vi "Sudo Wrapper.vi"(7 "Install LV Data":T1={"SSH Session"=refnum, "Status Log"="", "Detailed Log"="", "Credentials"={"Hostname or IP"="192.168.7.2", "Username"="root", "Password"=""}, "Target Info"={"OS Version"="", "CPU"="", "Systemd Version"="", "Internet Access"=FALSE, "Device Type"="", "LV Installed Ver"="", "LV Available Ver"="", "LV Upgrade Available"=FALSE, "Hostname"="", "NIC Info"=[]}, "Reboot Required?"=FALSE}, 9 "comand string":string, 11 "echo string":string) -> (3 "combined command string":string)   [LabVIEW 2020, in "LMH-LINX.lvlib"]
uses:
  LMH-LINX.lvlib
  Target Management/Install LV Data.ctl
  Target Management/Target Info.ctl
  Target Management/NIC Info.ctl
  Target Management/NIC Mode.ctl
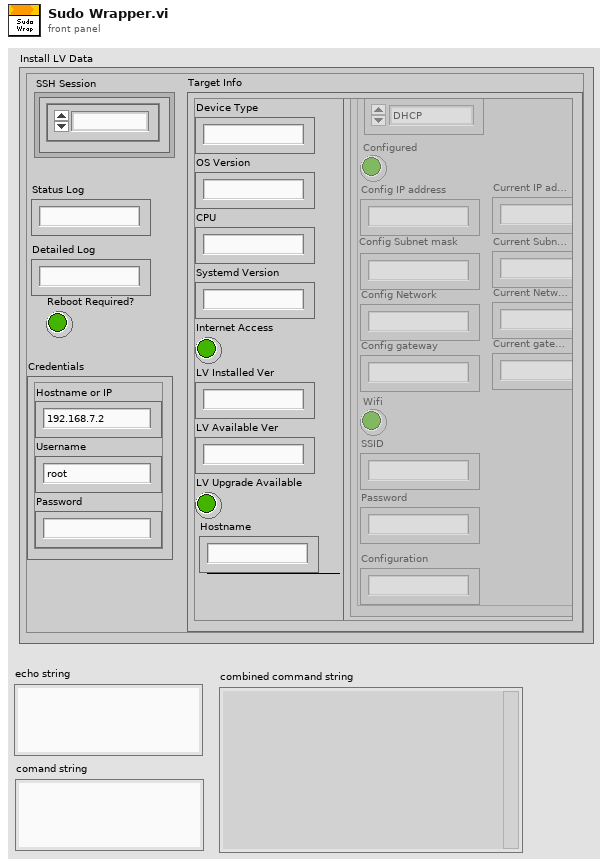
[diagram p1: front panel]
types:
  T1 = typedef "LMH-LINX.lvlib/Install LV Data.ctl" = cluster{"SSH Session":refnum<k1>, "Status Log":string, "Detailed Log":string, "Credentials":cluster{"Hostname or IP":string, "Username":string, "Password":string}, "Target Info":T2, "Reboot Required?":bool}
  T2 = typedef "LMH-LINX.lvlib/Target Info.ctl" = cluster{"OS Version":string, "CPU":string, "Systemd Version":string, "Internet Access":bool, "Device Type":string, "LV Installed Ver":string, "LV Available Ver":string, "LV Upgrade Available":bool, "Hostname":string, "NIC Info":T3[]}
  T3 = typedef "LMH-LINX.lvlib/NIC Info.ctl" = cluster{"Name":string, "NIC Mode":T4, "Configured":bool, "Config IP address":string, "Config Subnet mask":string, "Config Network":string, "Config gateway":string, "Wifi":bool, "SSID":string, "Password":string, "Configuration":string, "Current IP address":string, "Current Subnet mask":string, "Current gateway":string, "Current Network":string}
  T4 = typedef "LMH-LINX.lvlib/NIC Mode.ctl" = enum16{"DHCP", "Static", "Loopback"}
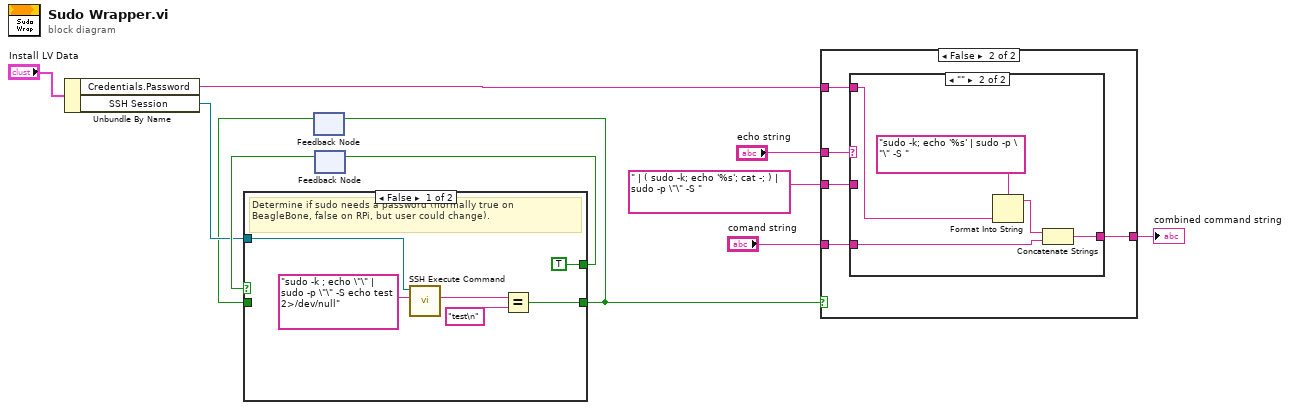
[diagram p0: block diagram]
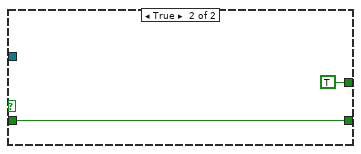
[diagram p2: hidden frame]
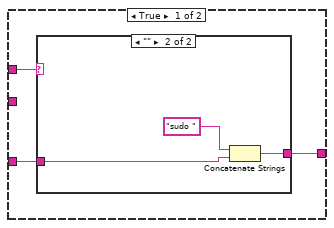
[diagram p3: hidden frame]
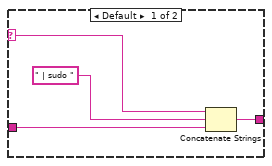
[diagram p4: hidden frame]
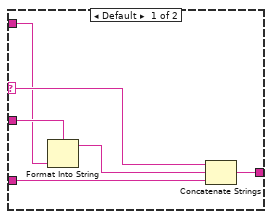
[diagram p5: hidden frame]
diagram:
  n1 = Unbundle By Name("Install LV Data") -> ("Credentials.Password"=w6:string, "SSH Session"=w3:refnum<k1>)
  n2 = feedback #1() -> (w2:bool)  [unwired: 1 in]
  n3 = feedback #2() -> (w5:bool)  [unwired: 1 in]
  n4 = case shown="False" w5 {
    tunnel: [TRUE TRUE] -> w4
    tunnel: w3 -> [w15 _]
    tunnel: [w12 w19] -> w1
    tunnel: w2 -> [_ w19]
    frame False {
      # "Determine if sudo needs a password (normally true on\nBeagleBone, false on RPi, but user could change)."
      n5 = call "SSH Execute Command.vi"("Command"="sudo -k ; echo \"\" | sudo -p \"\" -S echo test  2>/dev/null", "SSH Session"=w15) -> ("Std Out"=w14:string)  [unwired: 7 in, 2 out]
      n6 = Equal?(x=w14, y="test\n") -> (x = y?=w12:bool)
    }
    frame True {
    }
  }
  n7 = feedback-in #1(w1) -> ()
  n8 = feedback-in #2(w4) -> ()
  n9 = case shown="False" w1 {
    tunnel: "echo string" -> [w21 w34]
    tunnel: "comand string" -> [w20 w33]
    tunnel: [w22 w32] -> w9
    tunnel: " | ( sudo -k; echo '%s'; cat -; ) | sudo -p \"\" -S " ("Command") -> [_ w31]
    tunnel: w6 -> [_ w30]
    frame True {
      n10 = case shown="\"\"" w21 {
        selector: w21 -> [w25 _]
        tunnel: w20 -> [w26 w29]
        tunnel: [w24 w28] -> w22
        frame Default {
          n11 = Concatenate Strings(w25, " | sudo " ("Command"), w26) -> (w24:string)
        }
        frame "" {
          n12 = Concatenate Strings("sudo " ("Command"), w29) -> (w28:string)
        }
      }
    }
    frame False {
      n13 = case shown="\"\"" w34 {
        selector: w34 -> [w39 _]
        tunnel: w33 -> [w40 w45]
        tunnel: [w38 w44] -> w32
        tunnel: w31 -> [w37 _]
        tunnel: w30 -> [w35 w41]
        frame Default {
          n14 = Format Into String(format string=w37, w35) -> (resulting string=w36:string)  [unwired: 2 in, 1 out]
          n15 = Concatenate Strings(w39, w36, w40) -> (w38:string)
        }
        frame "" {
          n16 = Format Into String(format string="sudo -k; echo '%s' | sudo -p \"\" -S " ("Command"), w41) -> (resulting string=w43:string)  [unwired: 2 in, 1 out]
          n17 = Concatenate Strings(w43, w45) -> (w44:string)
        }
      }
    }
  }
  "combined command string" <- w9
